vi "AODScanner.vi"() -> ()   [LabVIEW 2011]
uses:
  AODAcq/AODAcq.lvclass
  <vilib>/DAQmx/write.llb/DAQmx Write (Analog DBL 1Chan 1Samp).vi
  <vilib>/DAQmx/read.llb/DAQmx Read (Analog Wfm 1Chan NSamp).vi
  <vilib>/DAQmx/miscellaneous.llb/DAQmx Fill In Error Info.vi
  <vilib>/Utility/error.llb/Error Cluster From Error Code.vi
  <vilib>/rvi/errors/niLvFpgaAdjustHostInterfaceError.vi
  <vilib>/rvi/interface/nirviMethod/nirviMethod.xnode
  FPGA_Control/AODRef.ctl
  FPGA Bitfiles/Acquisition_FPGATarget_AODControl(FPGA)_C1C38267.lvbitx
  FPGA_Control/AOD Control (FPGA).vi
  <vilib>/rvi/interface/nirviReadWriteControl/nirviReadWriteControl.xnode
  <vilib>/FPGAPlugInAG/PXIe-7965R/niLvFpga_ReadFifo_PXIe-7965R.vi
  <vilib>/rvi/errors/niLvFpgaMergeErrorWithErrorCode.vi
  NiFpgaLv.dll
panel:
  out "Temporal samples remaining":u32
  out "Motion samples remaining":u32
  out "Image samples remaining":u32
  out "Recording File":path
  out "Waveform Chart":waveform(dbl)(graph)
  out "Ephys":bool
  in  "TraceElements":u32=10000
  out "ScanProgress":dbl(slide) scale=0.0..1.0
  in  "Abort":bool
  out "Progress":dbl(slide) scale=0.0..1.0
  in  "SweepSettings":bool
  in  "stop":bool
  in  "Power":dbl(slide) min=0.0 max=5.0 step=0.1 scale=0.0..2.5
  out "Point Scanning":bool
  out "Volume Scanning":bool
  in  "Tab Control":enum32{"Setup", "Volume", "Traces", "Motion"}(tab)=enum."Volume"
  in  "Disp Volume":bool=TRUE
  in  "Save Volume":bool
  in  "Ephys":bool
  in  "Motion rate (Hz)":dbl
  in  "ClearPoints":bool
  in  "Scan Settings (um)":T1={"XStart"=-100, "XEnd"=100, "XNum"=250, "YStart"=-100, "YEnd"=100, "YNum"=250, "ZStart"=-50, "ZEnd"=50, "ZNum"=30}
  in  "Objective":enum16{"20x Olympus"}(ring)
  in  "Scan Time (s)":dbl=300.0
  in  "Volume Reps":i32=1 min=1 max=10000
  in  "Volume":bool
  in  "Scan":bool
  in  "Autoscale":bool
  out "Motion points":u32
  in  "MaxThreshold":dbl=1.0
  out "Number selected":u32
  in  "Number of cells":u32=200
  in  "Threshold":dbl=0.1
  in  "Contrast":dbl(slide)=700000.0 scale=0.0..0.002
  out "ImCh2":T2(plugin-control)
  out "ImCh1":T2(plugin-control)
  in  "Section":dbl min=0.0 max=0.0 step=1.0
  in  "Segment":bool
  out "Motion Increment":u32
  in  "DisplayVol":bool=TRUE
  in  "Offset":dbl(slide)=700000.0 scale=0.0..-2700000000.0
  out "Motion Ch1":T2(plugin-control)
  out "Ephys":waveform(dbl)[](graph)
  out "Traces":waveform(dbl)[](graph)
  in  "Down Rate":i32=500
  in  "Spacing":dbl=100.0
  in  "Decimate":bool
  in  "Baseline Offset":dbl
  out "Motion Ch2":T2(plugin-control)
  out "Finished":bool
  out "Stopped":bool
  out "AODAcq out":refnum<class "AODAcq.lvclass">
  in  "Debug":bool
  in  "GridPoints":u16=10
  out "Scan Settings":T1
  out "VolData":i32[][](array[numeric])
  in  "VolumeElements":u32=10000
  in  "Points":i32[][](array[numeric])
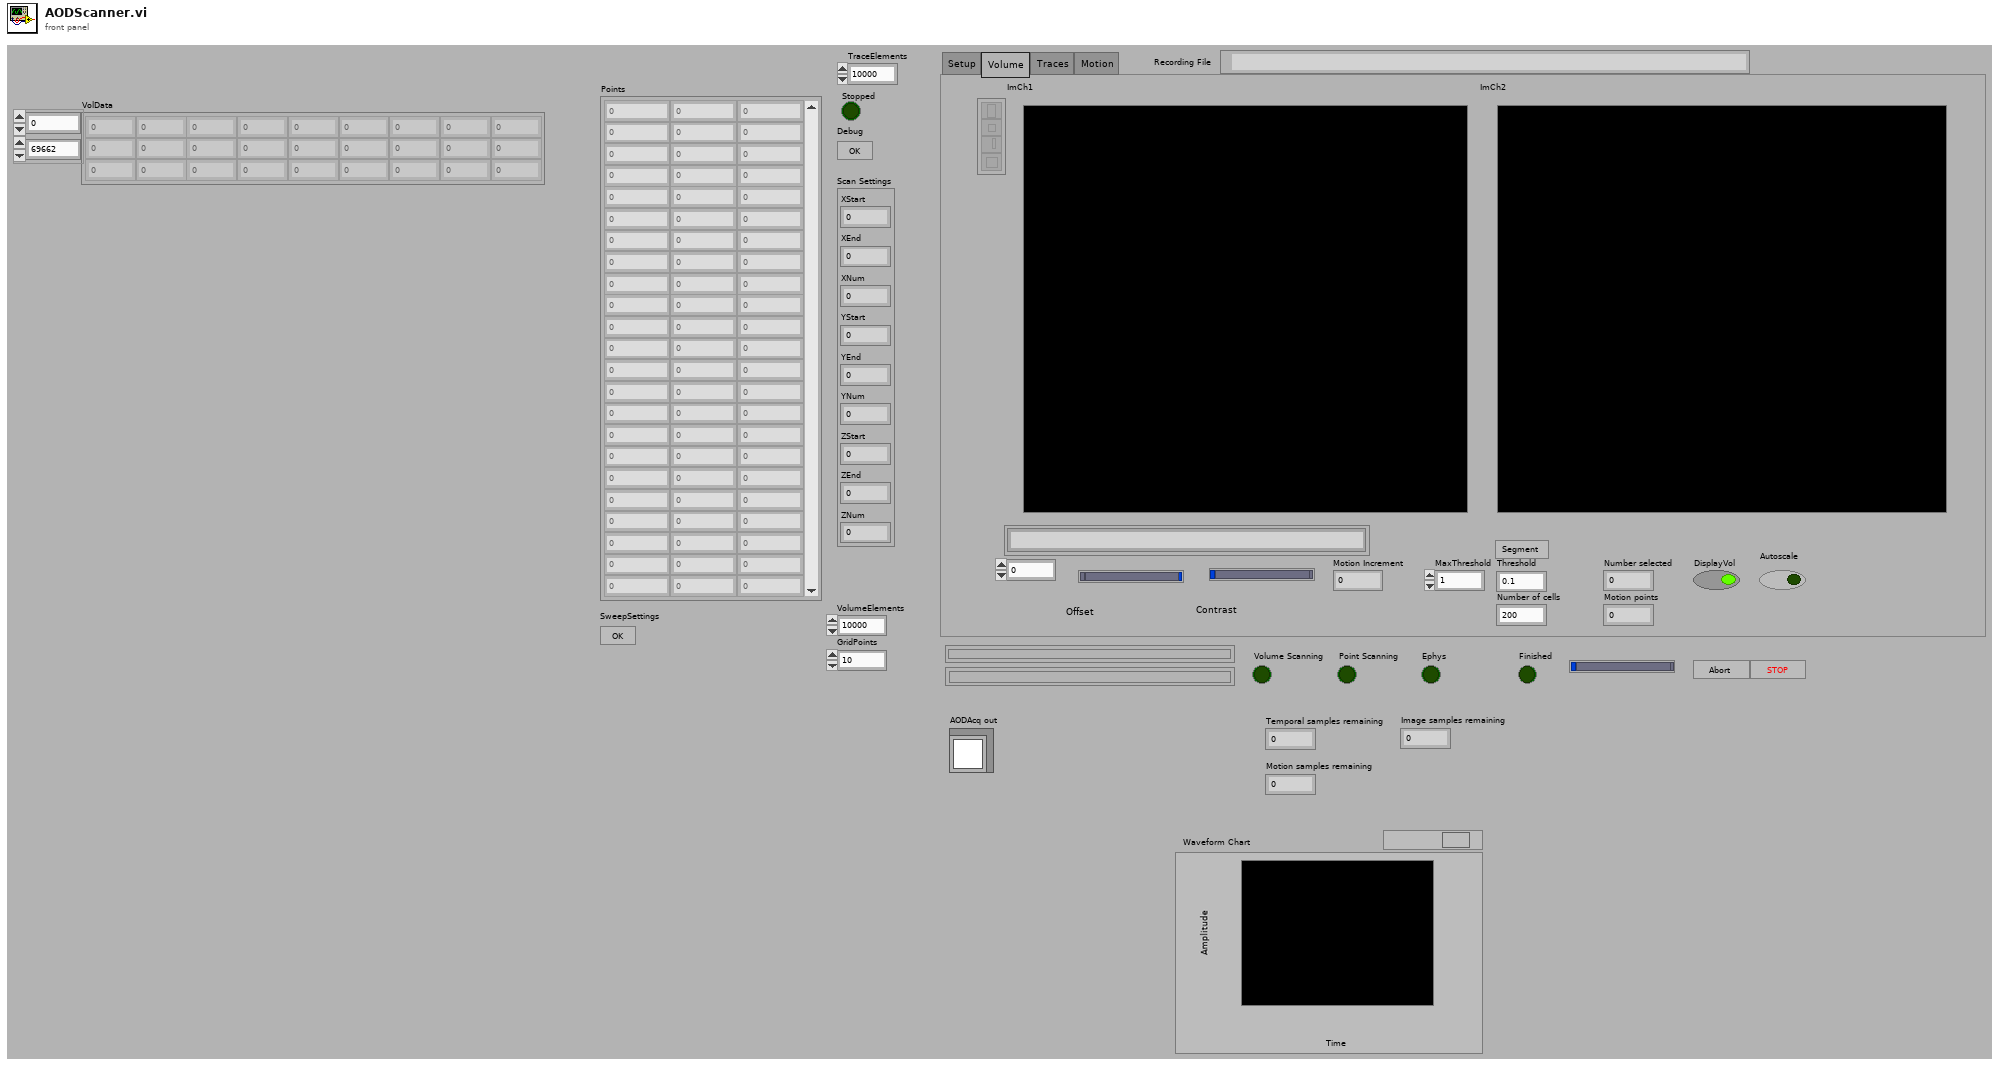
[diagram p1: front panel]
types:
  T1 = cluster{"XStart":i32, "XEnd":i32, "XNum":i32, "YStart":i32, "YEnd":i32, "YNum":i32, "ZStart":i32, "ZEnd":i32, "ZNum":i32}
  T2 = typedef "IMAQ Image.ctl" = refnum<image>
  T3 = typedef "Image Type" = u32
  T4 = cluster{"Global Rectangle":i32[], "Contours":cluster{"Contour Type":u32, "ROI Type":u32, "Points":i32[]}[]}
  T5 = cluster{"queue out":refnum<queue>, "queue out":refnum<queue>, "queue out":refnum<queue>}
  T6 = typedef "AODRef.ctl" = refnum<k20>
  T7 = cluster{"Global Rectangle":i32[], "Contours":cluster{"Contour Type":u32, "ROI Type":u32, "Points":i32[]}[]}[]
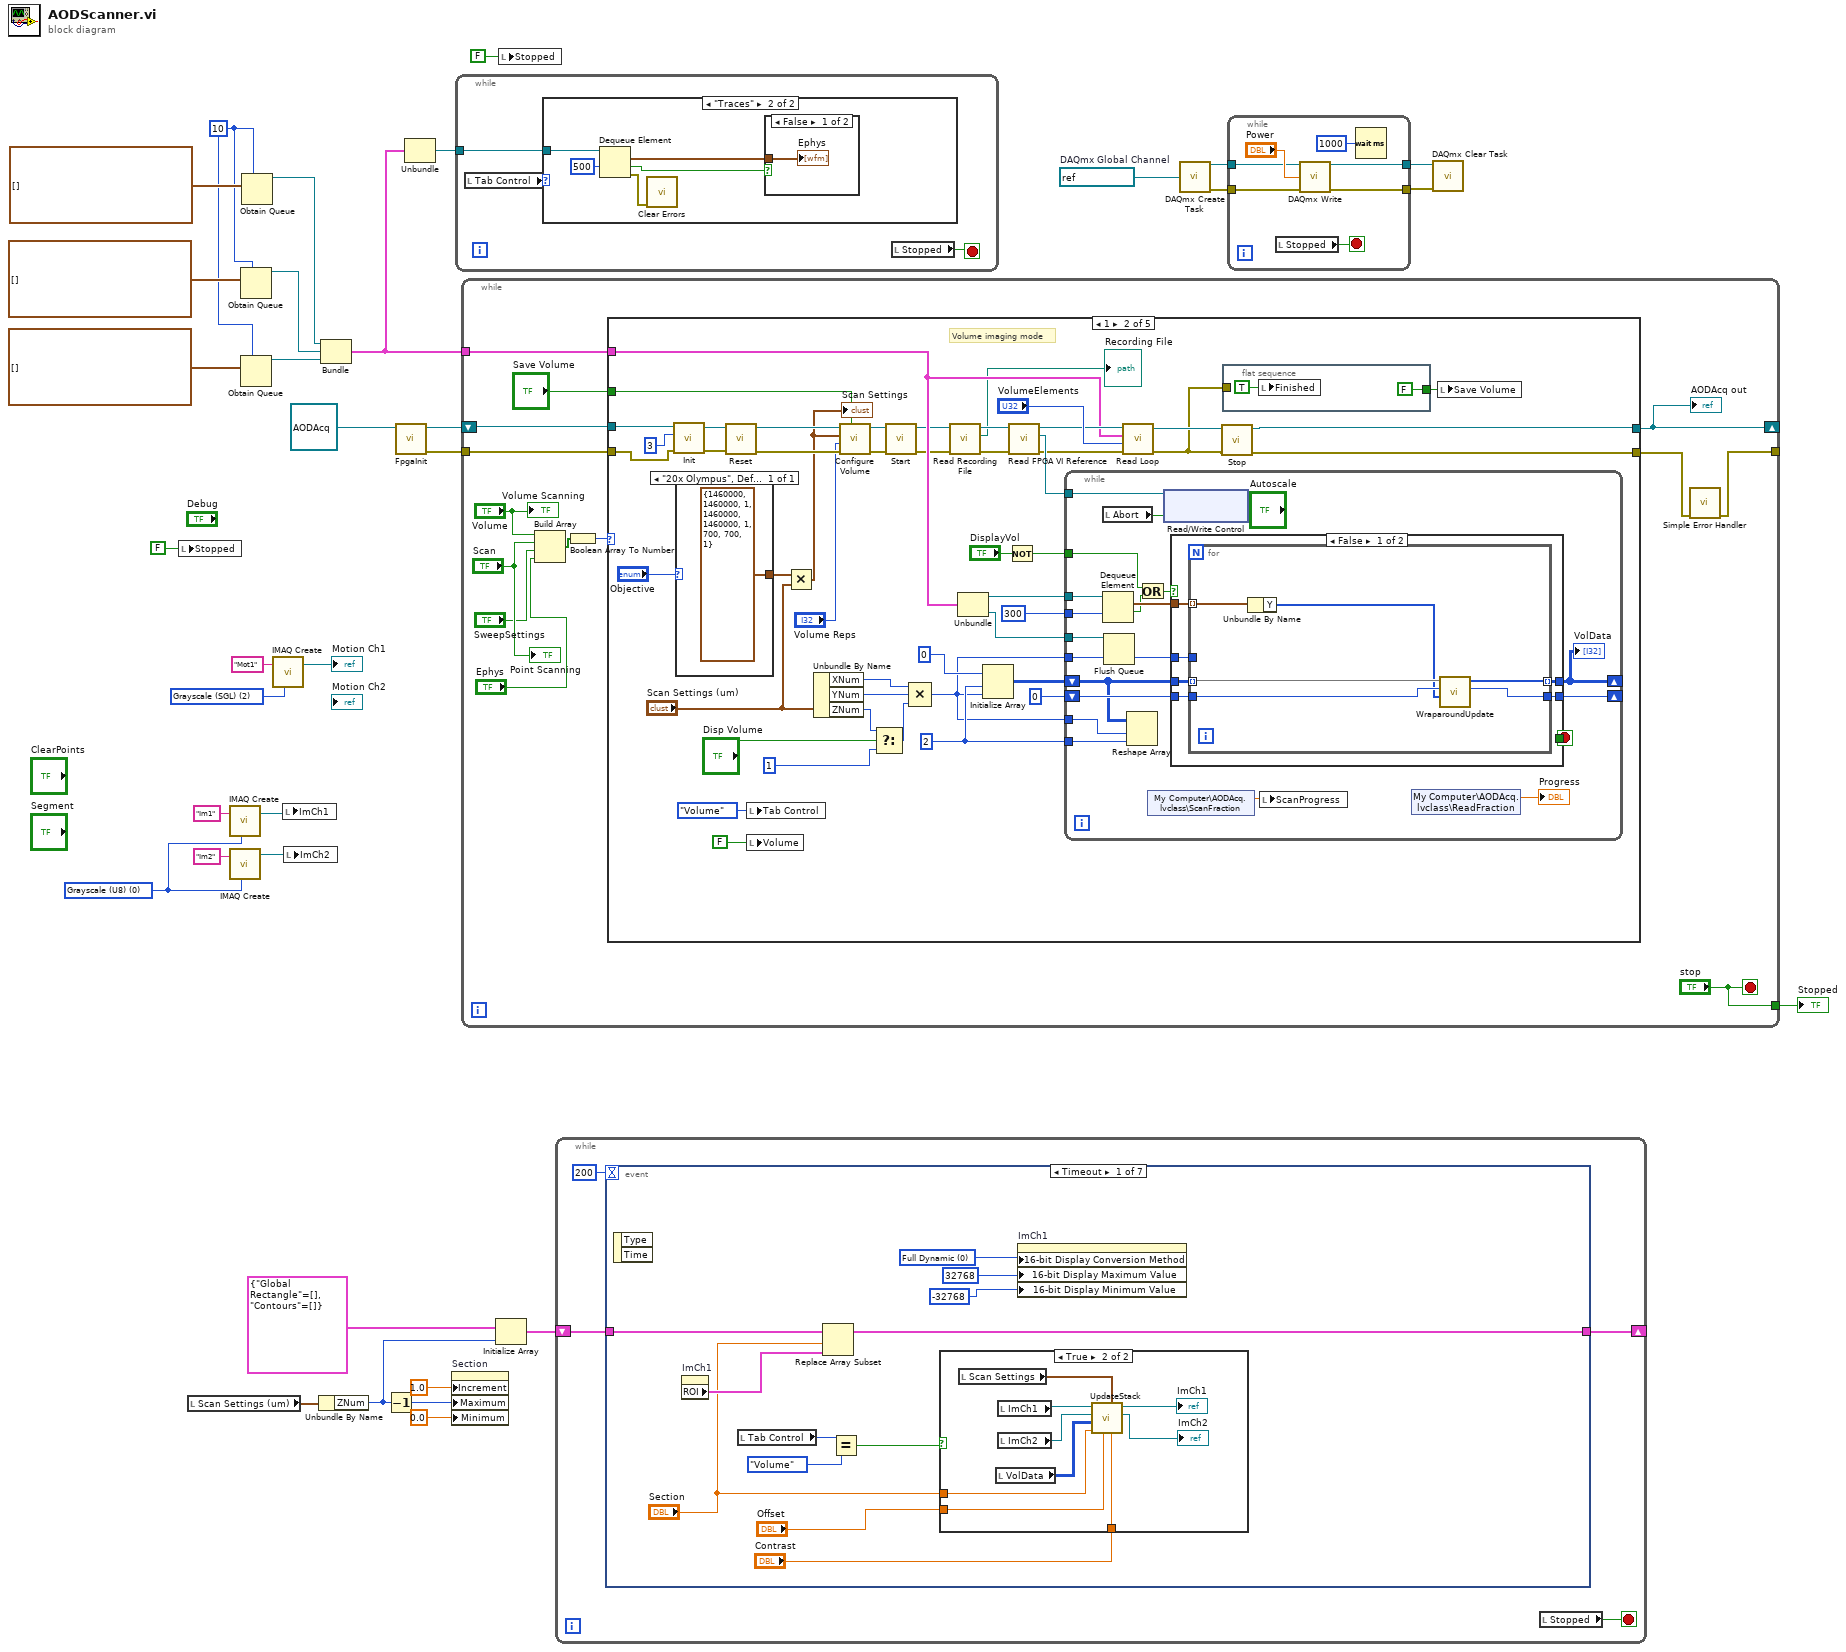
[diagram p0: block diagram]
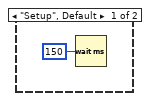
[diagram p2: hidden frame]
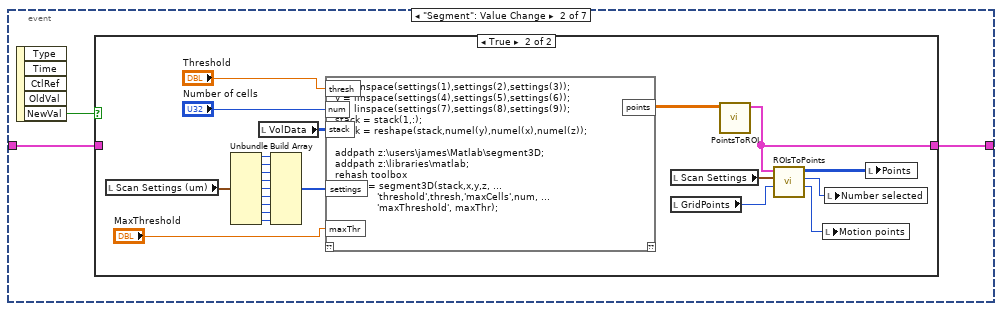
[diagram p5: hidden frame]
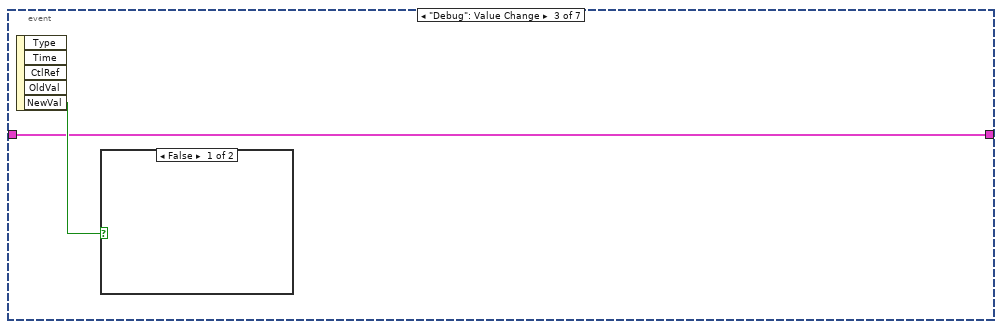
[diagram p7: hidden frame]
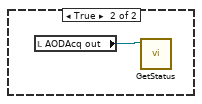
[diagram p8: hidden frame]
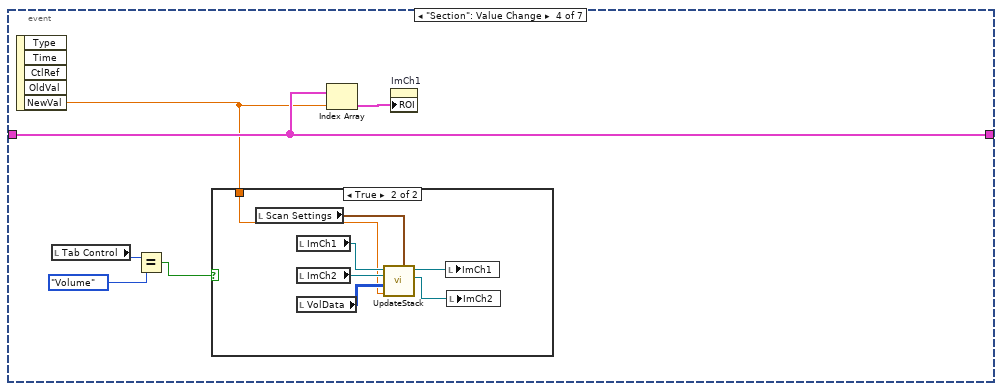
[diagram p9: hidden frame]
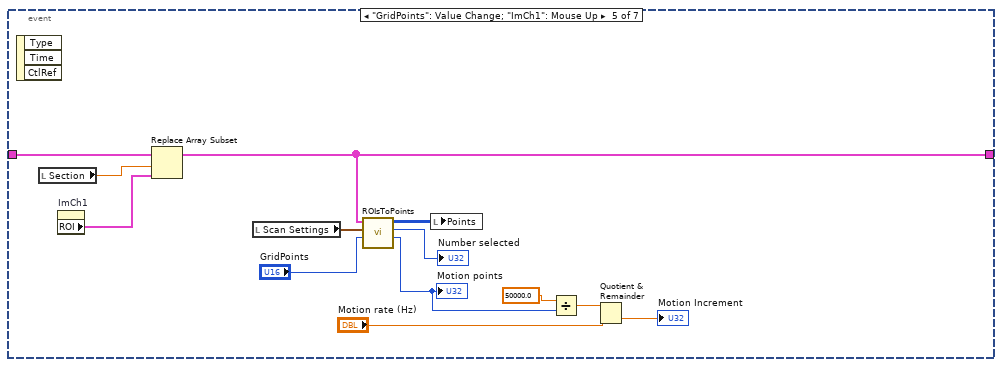
[diagram p11: hidden frame]
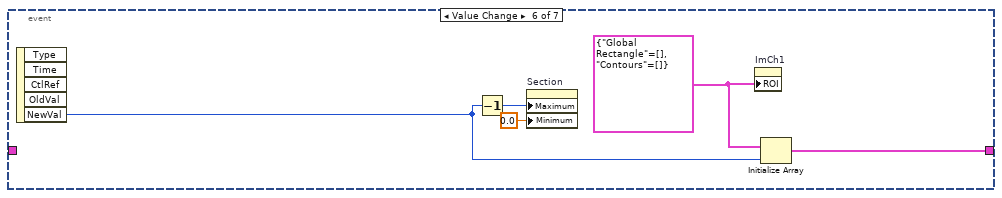
[diagram p12: hidden frame]
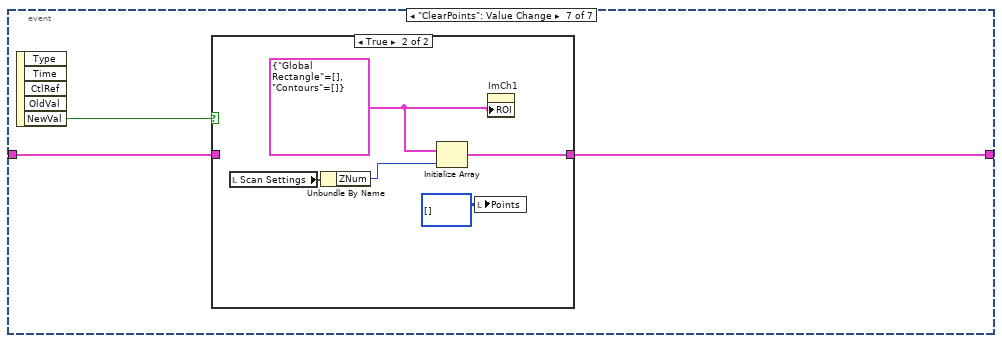
[diagram p13: hidden frame]
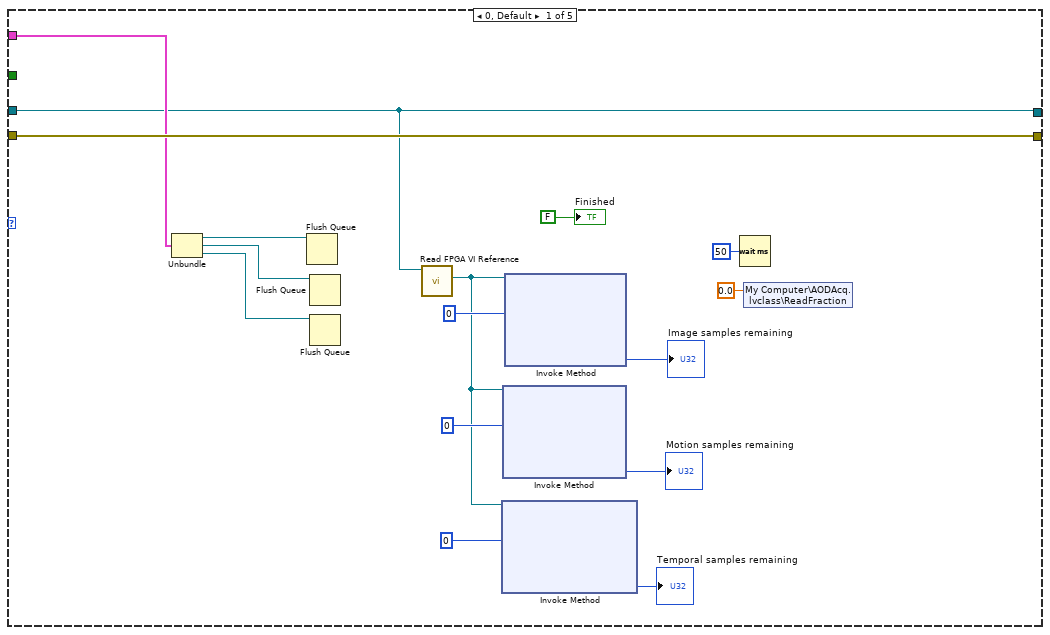
[diagram p15: hidden frame]
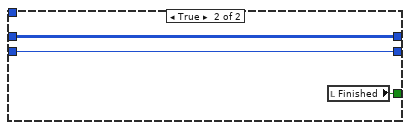
[diagram p16: hidden frame]
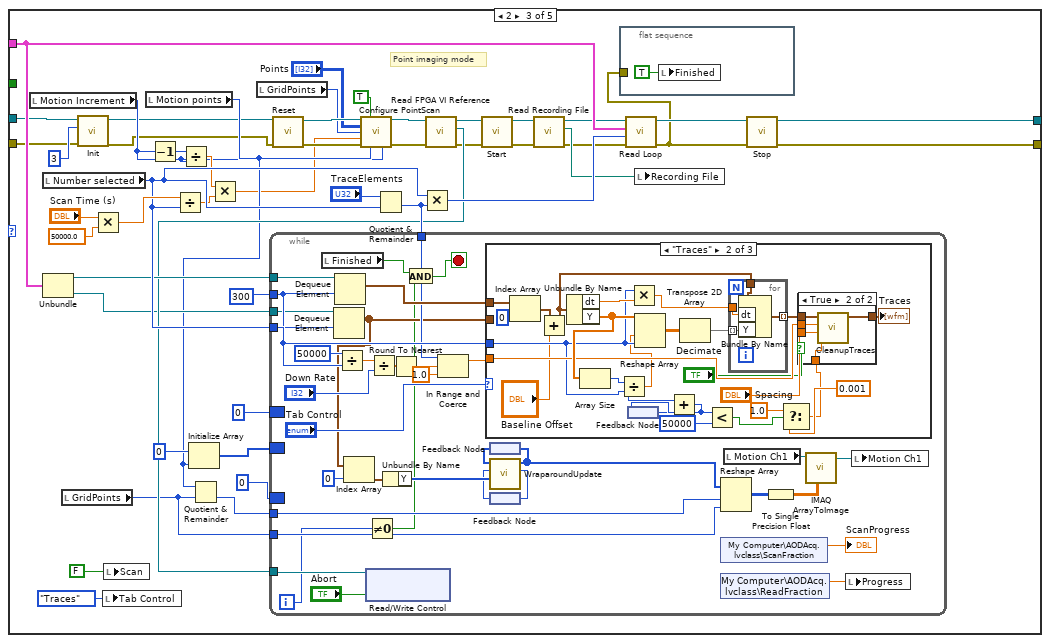
[diagram p17: hidden frame]
diagram:
  w1 = 10 ("max queue size (-1, unlimited)")
  w6 = T3 2 items=["Grayscale (U8)", "Grayscale (I16)", "Grayscale (SGL)", "Complex (CSG)", "RGB (U32)", "HSL (U32)", "RGB (U64)", "Grayscale (U16)"] ("Image Type")
  w18 = T3 0 items=["Grayscale (U8)", "Grayscale (I16)", "Grayscale (SGL)", "Complex (CSG)", "RGB (U32)", "HSL (U32)", "RGB (U64)", "Grayscale (U16)"] ("Image Type")
  w30 = refnum<k21> "AOD Gain"  # DAQmx Global Channel
  n1 = local write "Stopped"(FALSE ("Stopped")) -> ()
  n2 = local read "Scan Settings (um)"() -> (w23:T1)
  n3 = call "IMAQ Create"("Image Name"="Im1", "Image Type"=w18) -> ("New Image"=w32:T2)  [unwired: 3 in, 1 out]
  n4 = call "IMAQ Create"("Image Name"="Im2", "Image Type"=w18) -> ("New Image"=w31:T2)  [unwired: 3 in, 1 out]
  n5 = Obtain Queue(max queue size (-1, unlimited)=w1, element data type=waveform(dbl)[] []) -> (queue out=w13:refnum<queue>)  [unwired: 3 in, 2 out]
  n6 = Obtain Queue(max queue size (-1, unlimited)=w1, element data type=waveform(i32)[] []) -> (queue out=w11:refnum<queue>)  [unwired: 3 in, 2 out]
  n7 = Obtain Queue(max queue size (-1, unlimited)=w1, element data type=waveform(i32)[] []) -> (queue out=w12:refnum<queue>)  [unwired: 3 in, 2 out]
  n8 = call "IMAQ Create"("Image Name"="Mot1", "Image Type"=w6) -> ("New Image"=→"Motion Ch1":T2)  [unwired: 3 in, 1 out]
  n9 = local write "ImCh1"(w32) -> ()
  n10 = local write "ImCh2"(w31) -> ()
  n11 = Unbundle By Name(w23) -> ("ZNum"=w17:i32)
  n12 = Bundle("queue out"=w12, "queue out"=w13, "queue out"=w11) -> (w10:T5)  [unwired: 1 in]
  n13 = Decrement(x=w17) -> (x-1=w16:i32)
  n14 = call-dynamic "FpgaInit.vi"("AODAcq in"=refnum<class "AODAcq.lvclass"> refnum ("AODAcq.lvclass")) -> ("error out"=w4:errorcluster, "AODAcq out"=w3:refnum<class "AODAcq.lvclass">)  [unwired: 9 in]
  n15 = Unbundle(w10) -> ("queue out"=w9:refnum<queue>)  [unwired: 2 out]
  n16 = property on="Section" class="DigNum (strict)"("Increment"=1.0 ("Data Entry Limits:Increment"), "Maximum"=w16, "Minimum"=0.0 ("Data Entry Limits:Minimum")) -> ()  [unwired: 2 in, 2 out]
  n17 = while {
    tunnel: w9 -> [w38]
    stop <- w37 stop-if-true
    n18 = local read "Tab Control"() -> (w36:enum32{"Setup", "Volume", "Traces", "Motion"})
    n19 = case shown="\"Traces\"" w36 {
      tunnel: w38 -> [_ w44]
      frame "Setup", Default {
        n20 = Wait (ms)(milliseconds to wait=u32 150) -> ()  [unwired: 1 out]
      }
      frame "Traces" {
        n21 = Dequeue Element(queue=w44, timeout in ms (-1)=500) -> (element=w41:waveform(dbl)[], timed out?=w40:bool, error out=w42:errorcluster)  [unwired: 1 in, 1 out]
        n22 = call <vilib>:"Clear Errors.vi"("error in (no error)"=w42) -> ()  [unwired: 6 in, 1 out]
        n23 = case shown="False" w40 {
          tunnel: w41 -> [w45 _]
          frame False {
            "Ephys" <- w45
          }
          frame True {
          }
        }
      }
    }
    n24 = local read "Stopped"() -> (w37:bool)
  }
  n25 = while {
    shift-right: [w52] -> _
    shift-left: w3 -> [w59]
    tunnel: w10 -> [w53]
    tunnel: w4 -> [w58]
    tunnel: [w50] -> _
    tunnel: ["stop"] -> w27
    stop <- "stop" stop-if-true
    n26 = Build Array("Volume", "Scan", "SweepSettings", "Ephys") -> (w55:bool[])
    n27 = Boolean Array To Number(Boolean array=w55) -> (number=w54:u32)
    n28 = case shown="1" w54 {
      tunnel: w59 -> [w67 w88 w167 w285 w308]
      tunnel: w58 -> [w74 w87 w166 w284 _]
      tunnel: [w67 w100 w176 w289 w308] -> w52
      tunnel: [w74 w97 w175 w288 w307] -> w51
      tunnel: w53 -> [w71 w101 w197 _ w310]
      tunnel: "Save Volume" -> [_ w96 _ _ _]
      frame 0, Default {
        n29 = Unbundle(w71) -> ("queue out"=w70:refnum<queue>, "queue out"=w69:refnum<queue>, "queue out"=w68:refnum<queue>)
        n30 = Flush Queue(queue=w70) -> ()  [unwired: 1 in, 3 out]
        n31 = Flush Queue(queue=w69) -> ()  [unwired: 1 in, 3 out]
        n32 = Flush Queue(queue=w68) -> ()  [unwired: 1 in, 3 out]
        n33 = call-dynamic "Read FPGA VI Reference.vi"("AODAcq in"=w67) -> ("FPGA VI Reference"=w60:T6)  [unwired: 8 in, 2 out]
        n34 = xnode "Invoke Method"("FPGA VI Reference In"=w60, "Number of Elements"=u32 0) -> ("Elements Remaining"=→"Temporal samples remaining":u32)  [unwired: 2 in, 3 out]
        n35 = xnode "Invoke Method"("FPGA VI Reference In"=w60, "Number of Elements"=u32 0) -> ("Elements Remaining"=→"Motion samples remaining":u32)  [unwired: 2 in, 3 out]
        n36 = xnode "Invoke Method"("FPGA VI Reference In"=w60, "Number of Elements"=u32 0) -> ("Elements Remaining"=→"Image samples remaining":u32)  [unwired: 2 in, 3 out]
        n37 = Wait (ms)(milliseconds to wait=u32 50) -> ()  [unwired: 1 out]
        n38 = shared-variable "My Computer\\AODAcq.lvclass\\ReadFraction"(0.0 ("ReadFraction")) -> ()  [unwired: 1 in, 1 out]
        "Finished" <- FALSE ("Finished")
      }
      frame 1 {
        w79 = 2 ("dimension size")
        # "Volume imaging mode"
        n39 = call-dynamic "Init.vi"("error in (no error)"=w87, "Channel"=i16 3, "AODAcq in"=w88) -> ("error out"=w86:errorcluster, "AODAcq out"=w85:refnum<class "AODAcq.lvclass">)  [unwired: 7 in]
        n40 = case shown="\"20x Olympus\", Default" "Objective" {
          tunnel: [T1 {"XStart"=1460000, "XEnd"=1460000, "XNum"=1, "YStart"=1460000, "YEnd"=1460000, "YNum"=1, "ZStart"=700, "ZEnd"=700, "ZNum"=1} ("y")] -> w116
          frame "20x Olympus", Default {
          }
        }
        n41 = call-dynamic "Reset.vi"("error in (no error)"=w86, "AODAcq in"=w85) -> ("error out"=w122:errorcluster, "AODAcq out"=w123:refnum<class "AODAcq.lvclass">)  [unwired: 8 in]
        n42 = local write "Tab Control"(enum32{"Setup", "Volume", "Traces"}."Volume" ("Tab Control")) -> ()
        n43 = local write "Volume"(FALSE ("Volume")) -> ()
        n44 = Multiply(x=w116, y="Scan Settings (um)") -> (x*y=w119:T1)
        "Scan Settings" <- w119
        n45 = Unbundle By Name("Scan Settings (um)") -> ("XNum"=w118:i32, "YNum"=w117:i32, "ZNum"=w81:i32)
        n46 = call-dynamic "Configure Volume.vi"("Save"=w96, "error in (no error)"=w122, "NumReps"="Volume Reps", "Scan Settings"=w119, "AODAcq in"=w123) -> ("error out"=w104:errorcluster, "AODAcq out"=w105:refnum<class "AODAcq.lvclass">)  [unwired: 5 in]
        n47 = Select(t=w81, s="Disp Volume", f=u32 1) -> (s? t:f=w80:u32)
        n48 = call-dynamic "Start.vi"("error in (no error)"=w104, "AODAcq in"=w105) -> ("error out"=w92:errorcluster, "AODAcq out"=w94:refnum<class "AODAcq.lvclass">)  [unwired: 8 in]
        n49 = Compound Arithmetic op=MULTIPLY(w118, w117, w80) -> (w78:u32)
        n50 = call-dynamic "Read Recording File.vi"("error in (no error)"=w92, "AcquistionObject in"=w94) -> ("error out"=w91:errorcluster, "Recording File"=→"Recording File":path, "AcquistionObject out"=w93:refnum<class "AODAcq.lvclass">)  [unwired: 7 in]
        n51 = Unbundle(w101) -> ("queue out"=w109:refnum<queue>, "queue out"=w106:refnum<queue>)  [unwired: 1 out]
        n52 = Initialize Array(0, w79, w78) -> (w115:i32[][])
        n53 = Not(x="DisplayVol") -> (.not. x?=w76:bool)
        n54 = call-dynamic "Read FPGA VI Reference.vi"("error in (no error)"=w91, "AODAcq in"=w93) -> ("error out"=w102:errorcluster, "FPGA VI Reference"=w108:T6, "AODAcq out"=w103:refnum<class "AODAcq.lvclass">)  [unwired: 7 in]
        n55 = while {
          tunnel: w109 -> [w144]
          shift-right: [w140] -> _
          shift-left: w115 -> [w129]
          shift-right: [w141] -> _
          shift-left: 0 -> [w142]
          tunnel: w78 -> [w139]
          tunnel: 300 ("timeout in ms (-1)") -> [w138]
          tunnel: w108 -> [w135]
          tunnel: w106 -> [w133]
          tunnel: w79 -> [w131]
          tunnel: w78 -> [w130]
          tunnel: w76 -> [w126]
          stop <- w136 stop-if-true
          n56 = local read "Abort"() -> (w132:bool)
          n57 = Dequeue Element(queue=w144, timeout in ms (-1)=w138) -> (element=w143:waveform(i32)[], timed out?=w128:bool)  [unwired: 1 in, 2 out]
          n58 = Flush Queue(queue=w133) -> ()  [unwired: 1 in, 3 out]
          n59 = Reshape Array(w129, w130, w131) -> ()  [unwired: 1 out]
          n60 = Or(x=w126, y=w128) -> (x .or. y?=w127:bool)
          n61 = shared-variable "My Computer\\AODAcq.lvclass\\ScanFraction"() -> (w134:dbl)  [unwired: 1 in, 1 out]
          n62 = xnode "Read/Write Control"("FPGA VI Reference In"=w135, "Control.Abort"=w132) -> ()  [unwired: 1 in, 2 out]
          n63 = case shown="False" w127 {
            tunnel: w129 -> [w150 w159]
            tunnel: w143 -> [w149 _]
            tunnel: w142 -> [w148 w158]
            tunnel: [w147 w158] -> w141
            tunnel: [w146 w159] -> w140
            tunnel: w139 -> [w145 _]
            tunnel: [_ w157] -> w136
            frame False {
              n64 = for {
                tunnel: w150 -> [w154] mode=indexing
                tunnel: w149 -> [w156] mode=indexing
                tunnel: [w155] -> w146 mode=indexing
                tunnel: w148 -> [w152]
                tunnel: [w153] -> w147
                tunnel: w145 -> [_]
                n65 = Unbundle By Name(w156) -> ("Y"=w151:i32[])
                n66 = call "WraparoundUpdate.vi"("Data"=w151, "Location"=w152, "Accumulator"=w154) -> ("NewLocation"=w153:u32, "Accumulated"=w155:i32[])  [unwired: 7 in]
              }
            }
            frame True {
              n67 = local read "Finished"() -> (w157:bool)
            }
          }
          "VolData" <- w140
          n68 = local write "ScanProgress"(w134) -> ()
          n69 = shared-variable "My Computer\\AODAcq.lvclass\\ReadFraction"() -> (→"Progress":dbl)  [unwired: 1 in, 1 out]
        }
        n70 = call-dynamic "Read Loop.vi"("error in (no error)"=w102, "ReadElements"="VolumeElements", "Queues"=w101, "AODAcq in"=w103) -> ("error out"=w98:errorcluster, "AODAcq out"=w99:refnum<class "AODAcq.lvclass">)  [unwired: 6 in]
        n71 = call-dynamic "Stop.vi"("error in (no error)"=w98, "AODAcq in"=w99) -> ("error out"=w97:errorcluster, "AODAcq out"=w100:refnum<class "AODAcq.lvclass">)  [unwired: 8 in]
        n72 = flat-sequence {
          tunnel: w98 -> [_]
          tunnel: [FALSE] -> w95
          frame #0 {
            n73 = local write "Finished"(TRUE ("Finished")) -> ()
          }
        }
        n74 = local write "Save Volume"(w95) -> ()
      }
      frame 2 {
        # "Point imaging mode"
        n75 = local read "Motion Increment"() -> (w179:u32)
        n76 = local read "Number selected"() -> (w199:u32)
        n77 = Unbundle(w197) -> ("queue out"=w196:refnum<queue>, "queue out"=w192:refnum<queue>)  [unwired: 1 out]
        n78 = local read "GridPoints"() -> (w190:u16)
        n79 = call-dynamic "Init.vi"("error in (no error)"=w166, "Channel"=i16 3, "AODAcq in"=w167) -> ("error out"=w164:errorcluster, "AODAcq out"=w165:refnum<class "AODAcq.lvclass">)  [unwired: 7 in]
        n80 = Multiply(x="Scan Time (s)", y=50000.0) -> (x*y=w204:dbl)
        n81 = local write "Tab Control"(enum32{"Setup", "Volume", "Traces"}."Traces" ("Tab Control")) -> ()
        n82 = local write "Scan"(FALSE ("Scan")) -> ()
        n83 = local read "Motion points"() -> (w187:u32)
        n84 = Decrement(x=w179) -> (x-1=w181:u32)
        n85 = Divide(x=w204, y=w199) -> (x/y=w183:dbl)
        n86 = Divide(x=w181, y=w179) -> (x/y=w180:dbl)
        n87 = Initialize Array(0 ("element"), w187) -> (w188:i32[])
        n88 = Quotient & Remainder(x=w187, y=w190) -> (floor(x/y)=w191:u32)  [unwired: 1 out]
        n89 = Multiply(x=w180, y=w183) -> (x*y=w182:dbl)
        n90 = local read "GridPoints"() -> (w178:u16)
        n91 = call-dynamic "Reset.vi"("error in (no error)"=w164, "AODAcq in"=w165) -> ("error out"=w208:errorcluster, "AODAcq out"=w209:refnum<class "AODAcq.lvclass">)  [unwired: 8 in]
        n92 = call-dynamic "Configure PointScan.vi"("AODAcq in"=w209, "Save"=TRUE ("Save Volume"), "Points"="Points", "GridSize"=w178, "Reps"=w182, "error in (no error)"=w208, "Motion Points"=w187, "Motion Increment"=w179) -> ("AODAcq out"=w194:refnum<class "AODAcq.lvclass">, "error out"=w195:errorcluster)  [unwired: 6 in]
        n93 = Quotient & Remainder(x="TraceElements", y=w199) -> (floor(x/y)=w200:u32)  [unwired: 1 out]
        n94 = Multiply(x=w199, y=w200) -> (x*y=w198:u32)
        n95 = call-dynamic "Read FPGA VI Reference.vi"("error in (no error)"=w195, "AODAcq in"=w194) -> ("error out"=w174:errorcluster, "FPGA VI Reference"=w193:T6, "AODAcq out"=w173:refnum<class "AODAcq.lvclass">)  [unwired: 7 in]
        n96 = while {
          tunnel: w199 -> [w242]
          tunnel: 300 ("timeout in ms (-1)") -> [w232]
          tunnel: w200 -> [w237]
          tunnel: w196 -> [w235]
          tunnel: w193 -> [w234]
          tunnel: w192 -> [w215]
          tunnel: w191 -> [w224]
          tunnel: w190 -> [w223]
          border: w188 -> [_]
          border: 0 -> [_]
          border: 0 -> [_]
          i -> [w214]
          stop <- w211 stop-if-true
          n97 = local read "Finished"() -> (w212:bool)
          n98 = Dequeue Element(queue=w215, timeout in ms (-1)=w232) -> (element=w231:waveform(i32)[])  [unwired: 1 in, 3 out]
          n99 = Dequeue Element(queue=w235, timeout in ms (-1)=w232) -> (element=w246:waveform(i32)[])  [unwired: 1 in, 3 out]
          n100 = Divide(x=50000, y=w242) -> (x/y=w241:dbl)
          n101 = Index Array(array=w231, index=0) -> (element=w229:waveform(i32))
          n102 = xnode "Read/Write Control"("FPGA VI Reference In"=w234, "Control.Abort"="Abort") -> ()  [unwired: 1 in, 2 out]
          n103 = Not Equal To 0?(x=w214) -> (x != 0?=w213:bool)
          n104 = Divide(x=w241, y="Down Rate") -> (x/y=w244:dbl)
          n105 = Unbundle By Name(w229) -> ("Y"=w221:i32[])
          n106 = Round To Nearest(number=w244) -> (nearest integer value=w239:dbl)
          n107 = And(x=w212, y=w213) -> (x .and. y?=w211:bool)
          n108 = In Range and Coerce(upper limit=w237, x=w239, lower limit=1.0) -> (coerced(x)=w236:dbl)  [unwired: 1 out]
          n109 = case shown="\"Traces\"" "Tab Control" {
            tunnel: w242 -> [_ w262 _]
            tunnel: w246 -> [_ w268 _]
            tunnel: w236 -> [_ w265 _]
            tunnel: w231 -> [_ _ _]
            frame "Setup", Default {
            }
            frame "Traces" {
              n110 = Index Array(array=w268, index=0) -> (element=w249:waveform(i32))
              n111 = Add(x=w249, y="Baseline Offset") -> (x+y=w247:waveform(dbl))
              n112 = Unbundle By Name(w247) -> ("dt"=w270:dbl, "Y"=w267:dbl[])
              n113 = Array Size(array=w267) -> (size(s)=w257:i32)
              n114 = Divide(x=w257, y=w262) -> (x/y=w261:dbl)
              n115 = feedback #1() -> (w256:i32)
              n116 = Multiply(x=w262, y=w270) -> (x*y=w269:dbl)
              n117 = Reshape Array(w267, w261, w262) -> (w260:dbl[][])
              n118 = Add(x=w257, y=w256) -> (x+y=w252:i32)
              n119 = feedback-in #1(w252) -> ()
              n120 = Transpose 2D Array(2D array=w260) -> (transposed array=w259:dbl[][])
              n121 = Less?(x=w252, y=50000) -> (x < y?=w250:bool)
              n122 = for {
                tunnel: w269 -> [w281]
                tunnel: w247 -> [w280]
                tunnel: [w279] -> w264 mode=indexing
                tunnel: w259 -> [w278] mode=indexing
                n123 = Bundle By Name(cluster=w280, "dt"=w281, "Y"=w278) -> (w279:waveform(dbl))
              }
              n124 = Select(t=1.0, s=w250, f=0.001 ("Baseline Rate")) -> (s? t:f=w253:dbl)
              n125 = case shown="True" "Decimate" {
                tunnel: "Spacing" -> [_ w277]
                tunnel: w265 -> [_ w276]
                tunnel: w264 -> [w272 w275]
                tunnel: [w272 w274] -> w263
                tunnel: w253 -> [_ w273]
                frame False {
                }
                frame True {
                  n126 = call "CleanupTraces.vi"("Baseline Rate"=w273, "Spacing"=w277, "decimating factor"=w276, "Traces in"=w275) -> ("Traces out"=w274:waveform(dbl)[])  [unwired: 7 in]
                }
              }
              "Traces" <- w263
            }
            frame "Motion" {
            }
          }
          n127 = feedback #2() -> (w220:i32[])
          n128 = feedback #3() -> (w218:u32)
          n129 = call "WraparoundUpdate.vi"("Data"=w221, "Location"=w218, "Accumulator"=w220) -> ("NewLocation"=w219:u32, "Accumulated"=w217:i32[])  [unwired: 7 in]
          n130 = feedback-in #2(w217) -> ()
          n131 = feedback-in #3(w219) -> ()
          n132 = Reshape Array(w217, w224, w223) -> (w227:i32[][])
          n133 = shared-variable "My Computer\\AODAcq.lvclass\\ScanFraction"() -> (→"ScanProgress":dbl)  [unwired: 1 in, 1 out]
          n134 = shared-variable "My Computer\\AODAcq.lvclass\\ReadFraction"() -> (w225:dbl)  [unwired: 1 in, 1 out]
          n135 = local read "Motion Ch1"() -> (w226:T2)
          n136 = To Single Precision Float(number=w227) -> (single precision float=w222:sgl[][])
          n137 = call "IMAQ ArrayToImage"("Image Pixels (Float)"=w222, "Image"=w226) -> ("Image Out"=w228:T2)  [unwired: 8 in, 1 out]
          n138 = local write "Progress"(w225) -> ()
          n139 = local write "Motion Ch1"(w228) -> ()
        }
        n140 = call-dynamic "Start.vi"("error in (no error)"=w174, "AODAcq in"=w173) -> ("error out"=w170:errorcluster, "AODAcq out"=w172:refnum<class "AODAcq.lvclass">)  [unwired: 8 in]
        n141 = call-dynamic "Read Recording File.vi"("error in (no error)"=w170, "AcquistionObject in"=w172) -> ("error out"=w162:errorcluster, "Recording File"=w169:path, "AcquistionObject out"=w171:refnum<class "AODAcq.lvclass">)  [unwired: 7 in]
        n142 = flat-sequence {
          tunnel: w161 -> [_]
          frame #0 {
            n143 = local write "Finished"(TRUE ("Finished")) -> ()
          }
        }
        n144 = call-dynamic "Read Loop.vi"("error in (no error)"=w162, "ReadElements"=w198, "Queues"=w197, "AODAcq in"=w171) -> ("error out"=w161:errorcluster, "AODAcq out"=w177:refnum<class "AODAcq.lvclass">)  [unwired: 6 in]
        n145 = local write "Recording File"(w169) -> ()
        n146 = call-dynamic "Stop.vi"("error in (no error)"=w161, "AODAcq in"=w177) -> ("error out"=w175:errorcluster, "AODAcq out"=w176:refnum<class "AODAcq.lvclass">)  [unwired: 8 in]
      }
      frame 4 {
        n147 = call-dynamic "Reset.vi"("error in (no error)"=w284, "AODAcq in"=w285) -> ("error out"=w283:errorcluster, "AODAcq out"=w282:refnum<class "AODAcq.lvclass">)  [unwired: 8 in]
        n148 = call-dynamic "Read FPGA VI Reference.vi"("error in (no error)"=w283, "AODAcq in"=w282) -> ("error out"=w291:errorcluster, "FPGA VI Reference"=w292:T6, "AODAcq out"=w290:refnum<class "AODAcq.lvclass">)  [unwired: 7 in]
        n149 = flat-sequence {
          tunnel: w292 -> [w295]
          tunnel: w291 -> [w293]
          tunnel: w290 -> [w294]
          tunnel: [w294] -> w287
          tunnel: [w293] -> w286
          tunnel: [w297] -> w288
          tunnel: [w296] -> w289
          tunnel: w287 -> [w299]
          tunnel: w286 -> [w298]
          frame #0 {
            n150 = call "SweepSettings.vi"("FPGA VI Reference Out"=w295) -> ()  [unwired: 11 in]
          }
          frame #1 {
            n151 = call-dynamic "GetStatus.vi"("error in (no error)"=w298, "AODAcq in"=w299) -> ("error out"=w297:errorcluster, "AODAcq out"=w296:refnum<class "AODAcq.lvclass">)  [unwired: 7 in, 1 out]
          }
        }
      }
      frame 8 {
        n152 = call "DAQ Assistant"() -> ("task out"=w311:refnum<k21>, "error out"=w306:errorcluster)  [unwired: 16 in, 2 out]
        n153 = local write "Tab Control"(enum32{"Setup", "Volume", "Traces", "Motion"}."Traces" ("Tab Control")) -> ()
        n154 = local write "Ephys"(FALSE ("Ephys")) -> ()
        n155 = Unbundle(w310) -> ("queue out"=w304:refnum<queue>)  [unwired: 2 out]
        n156 = while {
          tunnel: w311 -> [w320]
          tunnel: w304 -> [w319]
          tunnel: [w318] -> w309
          tunnel: w306 -> [w317]
          tunnel: [w315] -> w305
          tunnel: [FALSE ("Ephys")] -> w301
          stop <- w321 stop-if-true
          n157 = call-poly <vilib>:"DAQmx Read.vi"("task/channels in"=w320, "error in"=w317) -> ("task out"=w318:refnum<k21>, "data"=w313:waveform(dbl), "error out"=w316:errorcluster)  [unwired: 11 in]
          "Waveform Chart" <- w313
          n158 = Build Array(w313) -> (w312:waveform(dbl)[])
          n159 = local read "Abort"() -> (w321:bool)
          n160 = Enqueue Element(queue=w319, element=w312, error in (no error)=w316) -> (error out=w315:errorcluster)  [unwired: 1 in, 2 out]
        }
        "Ephys" <- w301
        n161 = local write "Ephys"(TRUE ("Ephys")) -> ()
        n162 = call <vilib>:"DAQmx Clear Task.vi"("task in"=w309, "error in"=w305) -> ("error out"=w307:errorcluster)  [unwired: 13 in]
      }
    }
    "AODAcq out" <- w52
    n163 = call <vilib>:"Simple Error Handler.vi"("error in (no error)"=w51) -> ("error out"=w50:errorcluster)  [unwired: 4 in, 4 out]
    "Volume Scanning" <- "Volume"
    "Point Scanning" <- "Scan"
  }
  "Stopped" <- w27
  n164 = Initialize Array(T4 {"Global Rectangle"=[], "Contours"=[]} ("ROI"), w17) -> (w21:T7)
  n165 = local write "Stopped"(FALSE ("Stopped")) -> ()
  n166 = while {
    shift-right: [w324] -> _
    shift-left: w21 -> [w325]
    stop <- w322 stop-if-true
    n167 = event shown="[0] Timeout" {
      selector: _ -> [_ _ _ _ _ _ _]
      dyn-events: _ -> [_ _ _ _ _ _ _]
      timeout: 200 -> [_ _ _ _ _ _ _]
      tunnel: w325 -> [w336 w348 w373 w380 w401 _ w407]
      tunnel: [w337 w347 w373 w380 w398 w406 w408] -> w324
      event Timeout {
        w331 = u32 0 items=["Full Dynamic", "Downshift", "Given Range", "90% Dynamic", "Given Percent Range"] ("16-bit Display Mapping:Conversion Method")
        n168 = event-data() -> ()  [unwired: 1 in, 2 out]
        n169 = property on="ImCh1" class="ImageControl"() -> ("ROI"=w335:T4)  [unwired: 2 in, 2 out]
        n170 = local read "Tab Control"() -> (w334:enum32{"Setup", "Volume", "Traces", "Motion"})
        n171 = Replace Array Subset(array=w336, new element=w335, index="Section") -> (w337:T7)
        n172 = Equal?(x=w334, y=enum32{"Setup", "Volume", "Traces"}."Volume") -> (x = y?=w332:bool)
        n173 = case shown="True" w332 {
          tunnel: "Section" -> [_ w340]
          tunnel: "Offset" -> [_ w339]
          tunnel: "Contrast" -> [_ w338]
          frame False {
          }
          frame True {
            n174 = local read "Scan Settings"() -> (w341:T1)
            n175 = local read "VolData"() -> (w342:i32[][])
            n176 = local read "ImCh1"() -> (w346:T2)
            n177 = local read "ImCh2"() -> (w345:T2)
            n178 = call "UpdateStack.vi"("Contrast"=w338, "Scan Settings"=w341, "Offset"=w339, "Section"=w340, "ImData"=w342, "Im2 2"=w345, "Im1 In"=w346) -> ("Im2 Out"=→"ImCh2":T2, "Im1 Out"=→"ImCh1":T2)  [unwired: 3 in]
          }
        }
        n179 = property on="ImCh1" class="ImageControl"("16-bit Display Conversion Method"=w331, "16-bit Display Maximum Value"=32768 ("16-bit Display Mapping:Maximum Value"), "16-bit Display Minimum Value"=-32768 ("16-bit Display Mapping:Maximum Value")) -> ()  [unwired: 2 in, 2 out]
      }
      event "Segment": Value Change {
        n180 = event-data() -> ("NewVal"=w349:bool)  [unwired: 1 in, 4 out]
        n181 = case shown="True" w349 {
          tunnel: w348 -> [w350 _]
          tunnel: [w350 w357] -> w347
          frame False {
          }
          frame True {
            n182 = local read "Scan Settings (um)"() -> (w372:T1)
            n183 = Unbundle(w372) -> ("XStart"=w371:i32, "XEnd"=w370:i32, "XNum"=w369:i32, "YStart"=w368:i32, "YEnd"=w367:i32, "YNum"=w366:i32, "ZStart"=w365:i32, "ZEnd"=w364:i32, "ZNum"=w363:i32)
            n184 = local read "VolData"() -> (w358:i32[][])
            n185 = Build Array(w371, w370, w369, w368, w367, w366, w365, w364, w363) -> (w362:i32[])
            n186 = script code="x = linspace(settings(1),settings(2),settings(3));\ny = linspace(settings(4),settings(5),settings(6));\nz = linspace(settings(7),settings(8),settings(9));\nstack = stack(1,:);\nstack = reshape(stack,numel(y),numel(x),numel(z));\n\naddpath z:\\users\\james\\Matlab\\segment3D;\naddpath z:\\libraries\\matlab;\nrehash toolbox\npoints = segment3D(stack,x,y,z, ...\n              'threshold',thresh,'maxCells',num, ...\n              'maxThreshold', maxThr);"("stack"=w358, "settings"=w362, "num"="Number of cells", "thresh"="Threshold", "maxThr"="MaxThreshold") -> ("points"=w359:cdb[][])  [unwired: 1 in, 1 out]
            n187 = local read "Scan Settings"() -> (w354:T1)
            n188 = local read "GridPoints"() -> (w353:u16)
            n189 = call "PointsToROI.vi"("Points"=w359) -> ("ROIs"=w357:T7)  [unwired: 10 in]
            n190 = call "ROIsToPoints.vi"("GridPoints"=w353, "Scan Settings"=w354, "ROI"=w357) -> ("Number of motion points"=w351:i32, "Number of points"=w355:i32, "Points"=w356:i32[][])  [unwired: 6 in]
            n191 = local write "Motion points"(w351) -> ()
            n192 = local write "Number selected"(w355) -> ()
            n193 = local write "Points"(w356) -> ()
          }
        }
      }
      event "Debug": Value Change {
        n194 = event-data() -> ("NewVal"=w374:bool)  [unwired: 1 in, 4 out]
        n195 = case shown="False" w374 {
          frame False {
          }
          frame True {
            n196 = local read "AODAcq out"() -> (w375:refnum<class "AODAcq.lvclass">)
            n197 = call-dynamic "GetStatus.vi"("AODAcq in"=w375) -> ()  [unwired: 8 in, 3 out]
          }
        }
      }
      event "Section": Value Change {
        n198 = event-data() -> ("NewVal"=w379:dbl)  [unwired: 1 in, 4 out]
        n199 = local read "Tab Control"() -> (w378:enum32{"Setup", "Volume", "Traces", "Motion"})
        n200 = Equal?(x=w378, y=enum32{"Setup", "Volume", "Traces"}."Volume") -> (x = y?=w376:bool)
        n201 = case shown="True" w376 {
          tunnel: w379 -> [_ w383]
          frame False {
          }
          frame True {
            n202 = local read "Scan Settings"() -> (w382:T1)
            n203 = local read "ImCh1"() -> (w386:T2)
            n204 = local read "ImCh2"() -> (w387:T2)
            n205 = local read "VolData"() -> (w388:i32[][])
            n206 = call "UpdateStack.vi"("Scan Settings"=w382, "Section"=w383, "ImData"=w388, "Im2 2"=w387, "Im1 In"=w386) -> ("Im2 Out"=w385:T2, "Im1 Out"=w384:T2)  [unwired: 5 in]
            n207 = local write "ImCh1"(w384) -> ()
            n208 = local write "ImCh2"(w385) -> ()
          }
        }
        n209 = Index Array(array=w380, index=w379) -> (element=w381:T4)
        n210 = property on="ImCh1" class="ImageControl"("ROI"=w381) -> ()  [unwired: 2 in, 2 out]
      }
      event "GridPoints": Value Change; "ImCh1": Mouse Up {
        n211 = event-data() -> ()  [unwired: 1 in, 3 out]
        n212 = local read "Section"() -> (w399:dbl)
        n213 = property on="ImCh1" class="ImageControl"() -> ("ROI"=w400:T4)  [unwired: 2 in, 2 out]
        n214 = Replace Array Subset(array=w401, new element=w400, index=w399) -> (w398:T7)
        n215 = local read "Scan Settings"() -> (w397:T1)
        n216 = call "ROIsToPoints.vi"("GridPoints"="GridPoints", "Scan Settings"=w397, "ROI"=w398) -> ("Number of motion points"=w392:i32, "Number of points"=→"Number selected":i32, "Points"=w395:i32[][])  [unwired: 6 in]
        "Motion points" <- w392
        n217 = local write "Points"(w395) -> ()
        n218 = Divide(x=50000.0, y=w392) -> (x/y=w391:dbl)
        n219 = Quotient & Remainder(x=w391, y="Motion rate (Hz)") -> (floor(x/y)=→"Motion Increment":dbl)  [unwired: 1 out]
      }
      event "Scan Settings (um).ZNum": Value Change {
        w405 = T4 {"Global Rectangle"=[], "Contours"=[]} ("ROI")
        n220 = event-data() -> ("NewVal"=w402:i32)  [unwired: 1 in, 4 out]
        n221 = Decrement(x=w402) -> (x-1=w403:i32)
        n222 = property on="Section" class="DigNum (strict)"("Maximum"=w403, "Minimum"=0.0 ("Data Entry Limits:Minimum")) -> ()  [unwired: 2 in, 2 out]
        n223 = property on="ImCh1" class="ImageControl"("ROI"=w405) -> ()  [unwired: 2 in, 2 out]
        n224 = Initialize Array(w405, w402) -> (w406:T7)
      }
      event "ClearPoints": Value Change {
        n225 = event-data() -> ("NewVal"=w409:bool)  [unwired: 1 in, 4 out]
        n226 = case shown="True" w409 {
          tunnel: [w410 w415] -> w408
          tunnel: w407 -> [w410 _]
          frame False {
          }
          frame True {
            w414 = T4 {"Global Rectangle"=[], "Contours"=[]} ("ROI")
            n227 = local read "Scan Settings"() -> (w413:T1)
            n228 = Unbundle By Name(w413) -> ("ZNum"=w412:i32)
            n229 = Initialize Array(w414, w412) -> (w415:T7)
            n230 = local write "Points"(i32[][] [] ("Points")) -> ()
            n231 = property on="ImCh1" class="ImageControl"("ROI"=w414) -> ()  [unwired: 2 in, 2 out]
          }
        }
      }
    }
    n232 = local read "Stopped"() -> (w322:bool)
  }
  n233 = call <vilib>:"DAQmx Create Task.vi"("global virtual channels"=w30) -> ("task out"=w29:refnum<k21>, "error out"=w28:errorcluster)  [unwired: 4 in, 9 out]
  n234 = while {
    tunnel: w29 -> [w421]
    tunnel: w28 -> [w420]
    tunnel: [w419] -> w26
    tunnel: [w418] -> w25
    stop <- w417 stop-if-true
    n235 = local read "Stopped"() -> (w417:bool)
    n236 = call-poly <vilib>:"DAQmx Write.vi"("task/channels in"=w421, "data"="Power", "error in"=w420) -> ("task out"=w419:refnum<k21>, "error out"=w418:errorcluster)  [unwired: 10 in, 1 out]
    n237 = Wait (ms)(milliseconds to wait=u32 1000) -> ()  [unwired: 1 out]
  }
  n238 = call <vilib>:"DAQmx Clear Task.vi"("task in"=w26, "error in"=w25) -> ()  [unwired: 13 in, 1 out]
